vi "GET_error_memory_error_log_error_input.vi"(4 "update_err_log":bool, 5 "update_err_input":bool, 6 "update_err_mem":bool, 7 "API Key":string="cheia04042025tema2restfulapi") -> (22 "body_error_log":string, 23 "get_error_memory":string, 24 "body_error_input":string, 25 "get_error_log_header":string, 26 "body_error_memory":string, 27 "get_error_input_header":string)   [LabVIEW 2024]
uses:
  <vilib>/httpClient/LabVIEWHTTPClient.lvlib
panel:
  out "error out get error input":errorcluster
  out "error out get error log":errorcluster
  out "error out get error memory":errorcluster
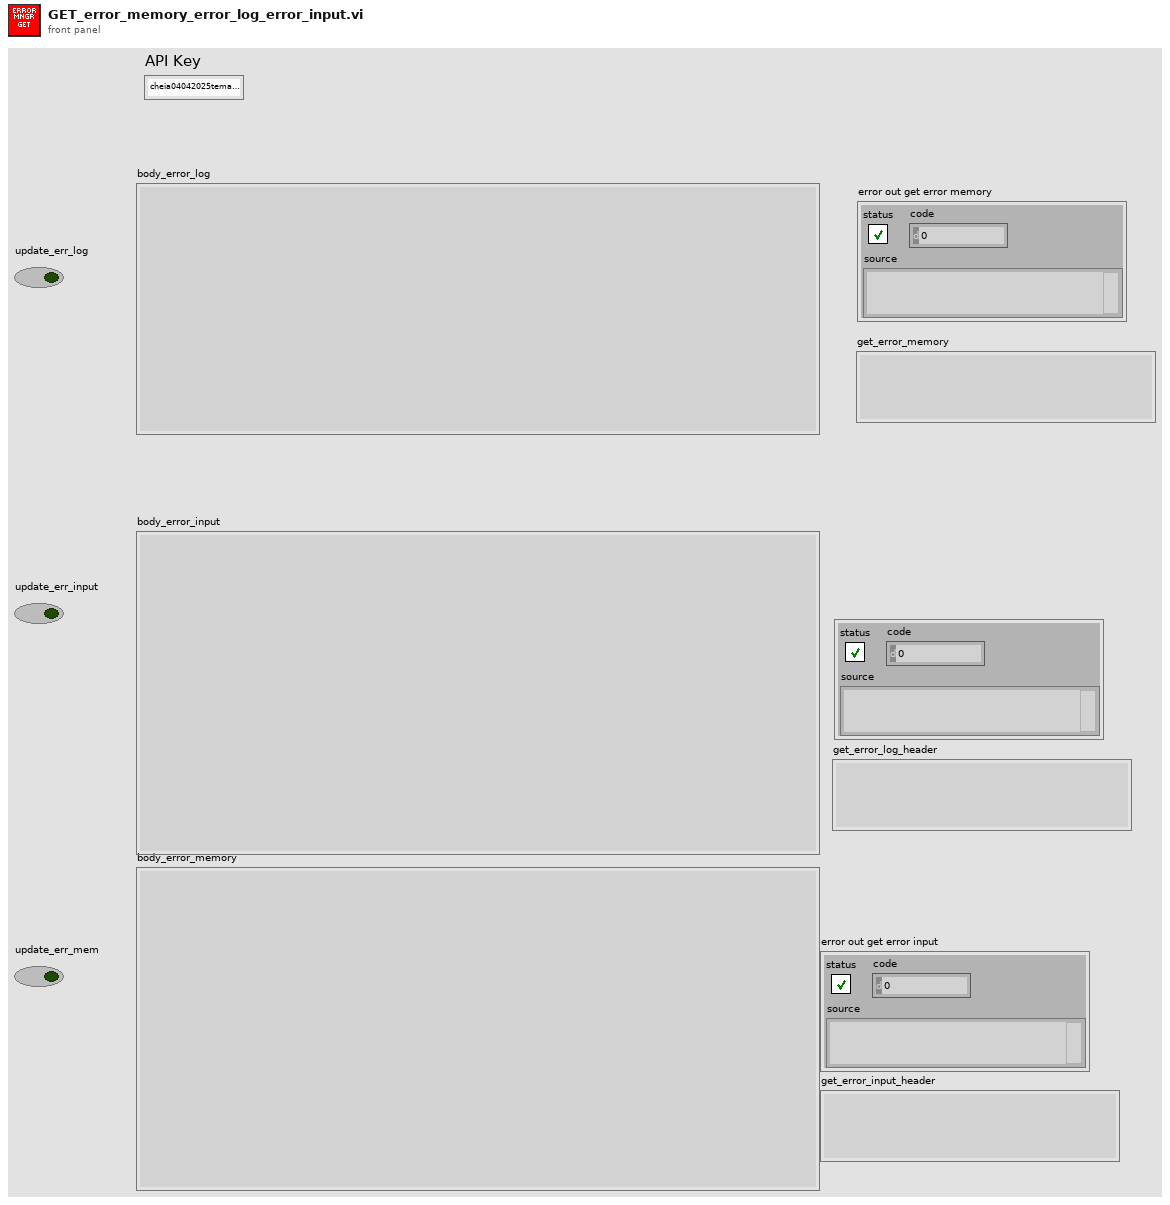
[diagram p1: front panel]
types:
  T1 = typedef "LabVIEWHTTPClient.lvlib/ClientHandle.ctl" = refnum<k1>
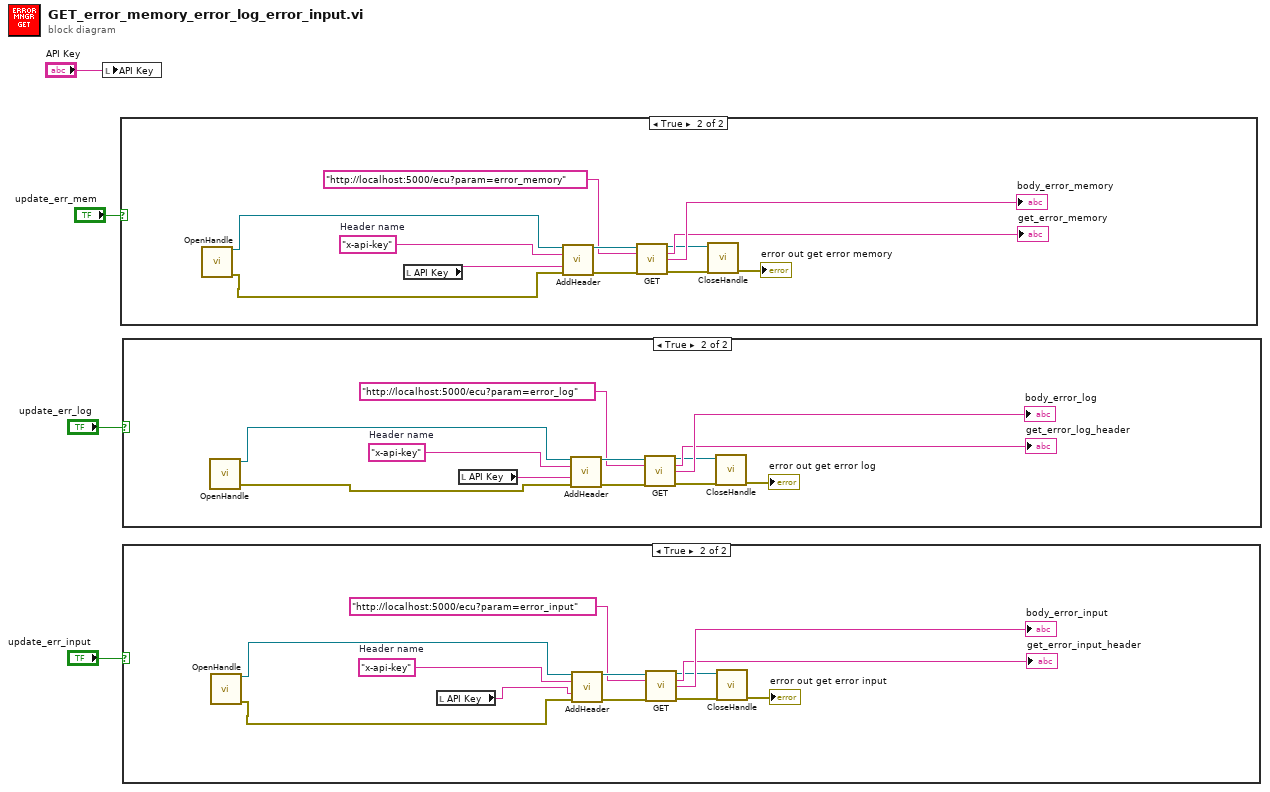
[diagram p0: block diagram]
diagram:
  n1 = local write "API Key"("API Key") -> ()
  n2 = case shown="True" "update_err_mem" {
    frame False {
    }
    frame True {
      w6 = "x-api-key"  # Header name
      n3 = call <vilib>:"OpenHandle.vi"() -> ("client handle out"=w8:T1, "error out"=w9:errorcluster)  [unwired: 14 in]
      n4 = local read "API Key"() -> (w5:string)
      n5 = call <vilib>:"AddHeader.vi"("client handle"=w8, "header"=w6, "value"=w5, "error in (no error)"=w9) -> ("client handle out"=w11:T1, "error out"=w10:errorcluster)  [unwired: 10 in]
      n6 = call <vilib>:"GET.vi"("client handle"=w11, "url"="http://localhost:5000/ecu?param=error_memory", "error in (no error)"=w10) -> ("client handle out"=w13:T1, "headers"=→"get_error_memory":string, "body"=→"body_error_memory":string, "error out"=w12:errorcluster)  [unwired: 9 in]
      n7 = call <vilib>:"CloseHandle.vi"("client handle"=w13, "error in (no error)"=w12) -> ("error out"=→"error out get error memory":errorcluster)  [unwired: 13 in]
    }
  }
  n8 = case shown="True" "update_err_log" {
    frame False {
    }
    frame True {
      w19 = "x-api-key"  # Header name
      n9 = call <vilib>:"OpenHandle.vi"() -> ("client handle out"=w21:T1, "error out"=w17:errorcluster)  [unwired: 14 in]
      n10 = local read "API Key"() -> (w18:string)
      n11 = call <vilib>:"AddHeader.vi"("client handle"=w21, "header"=w19, "value"=w18, "error in (no error)"=w17) -> ("client handle out"=w23:T1, "error out"=w22:errorcluster)  [unwired: 10 in]
      n12 = call <vilib>:"GET.vi"("client handle"=w23, "url"="http://localhost:5000/ecu?param=error_log", "error in (no error)"=w22) -> ("client handle out"=w25:T1, "headers"=→"get_error_log_header":string, "body"=→"body_error_log":string, "error out"=w24:errorcluster)  [unwired: 9 in]
      n13 = call <vilib>:"CloseHandle.vi"("client handle"=w25, "error in (no error)"=w24) -> ("error out"=→"error out get error log":errorcluster)  [unwired: 13 in]
    }
  }
  n14 = case shown="True" "update_err_input" {
    frame False {
    }
    frame True {
      w30 = "x-api-key"  # Header name
      n15 = call <vilib>:"OpenHandle.vi"() -> ("client handle out"=w32:T1, "error out"=w33:errorcluster)  [unwired: 14 in]
      n16 = local read "API Key"() -> (w29:string)
      n17 = call <vilib>:"AddHeader.vi"("client handle"=w32, "header"=w30, "value"=w29, "error in (no error)"=w33) -> ("client handle out"=w35:T1, "error out"=w34:errorcluster)  [unwired: 10 in]
      n18 = call <vilib>:"GET.vi"("client handle"=w35, "url"="http://localhost:5000/ecu?param=error_input", "error in (no error)"=w34) -> ("client handle out"=w37:T1, "headers"=→"get_error_input_header":string, "body"=→"body_error_input":string, "error out"=w36:errorcluster)  [unwired: 9 in]
      n19 = call <vilib>:"CloseHandle.vi"("client handle"=w37, "error in (no error)"=w36) -> ("error out"=→"error out get error input":errorcluster)  [unwired: 13 in]
    }
  }
